vi "Add Copyright.vi"(8 "error in (no error)":errorcluster, 9 "Delimiter":string, 10 "Copyright":string, 11 "Item in":refnum<class "Item.lvclass">) -> (0 "error out":errorcluster, 3 "Item out":refnum<class "Item.lvclass">)   [LabVIEW 2020, in "VI Properties Editor.lvlib" / "Item.lvclass"]
doc: "Adds <B>Copyright</B> to <B>Item in</B>."
uses:
  Item.lvclass
  Item.lvclass/Item.ctl
  VI Properties Editor.lvlib
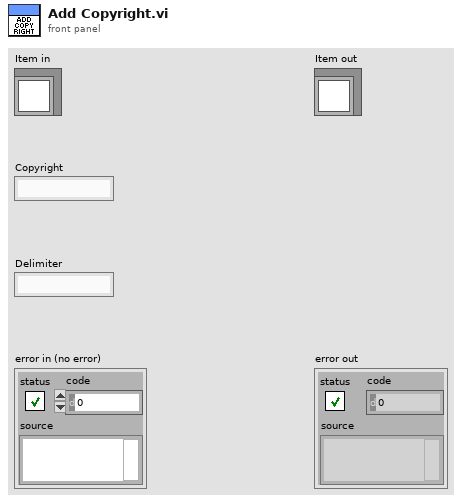
[diagram p1: front panel]
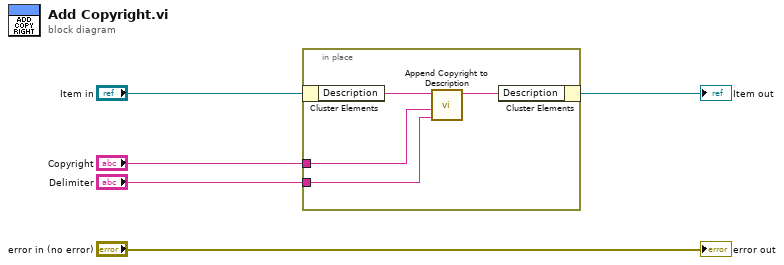
[diagram p0: block diagram]
diagram:
  n1 = in-place {
    in-place-border: "Copyright" -> [w7]
    in-place-border: "Delimiter" -> [w6]
    n2 = in-place-cluster #1("Item in") -> ("Description"=w9:string)
    n3 = call "Append Copyright to Description.vi"("Delimiter"=w6, "Copyright Text"=w7, "Description"=w9) -> ("Description out"=w8:string)  [unwired: 8 in]
    n4 = in-place-cluster #1("Description"=w8) -> (→"Item out":refnum<class "Item.lvclass">)
  }
  "error out" <- "error in (no error)"
